vi "WLAN_FrameAnalysis.vi"(8 "error in (no error)":errorcluster, 11 "input cluster":cluster{"t0":dbl, "dt":dbl, "Y":cdb[]}) -> (0 "error out":errorcluster, 1 "Constellation":cdb[](graph), 2 "Modulation parameter":T1, 3 "output bits":i8[](array[numeric]), 4 "Frequency offset":dbl, 5 "SIG valid?":bool)   [LabVIEW 2014]
panel:
  out "size(s) 3":i32
  out "size(s) 2":i32
  out "size(s)":i32
  out "Symbol numbers":i32
  out "encoded bit numbers":u32
  out "original bit numbers":u32
  out "Channel Esitimate":dbl[](graph)
  out "Frequency offset corrected signal":cluster{"t0":dbl, "dt":dbl, "Y":dbl[]}(graph)
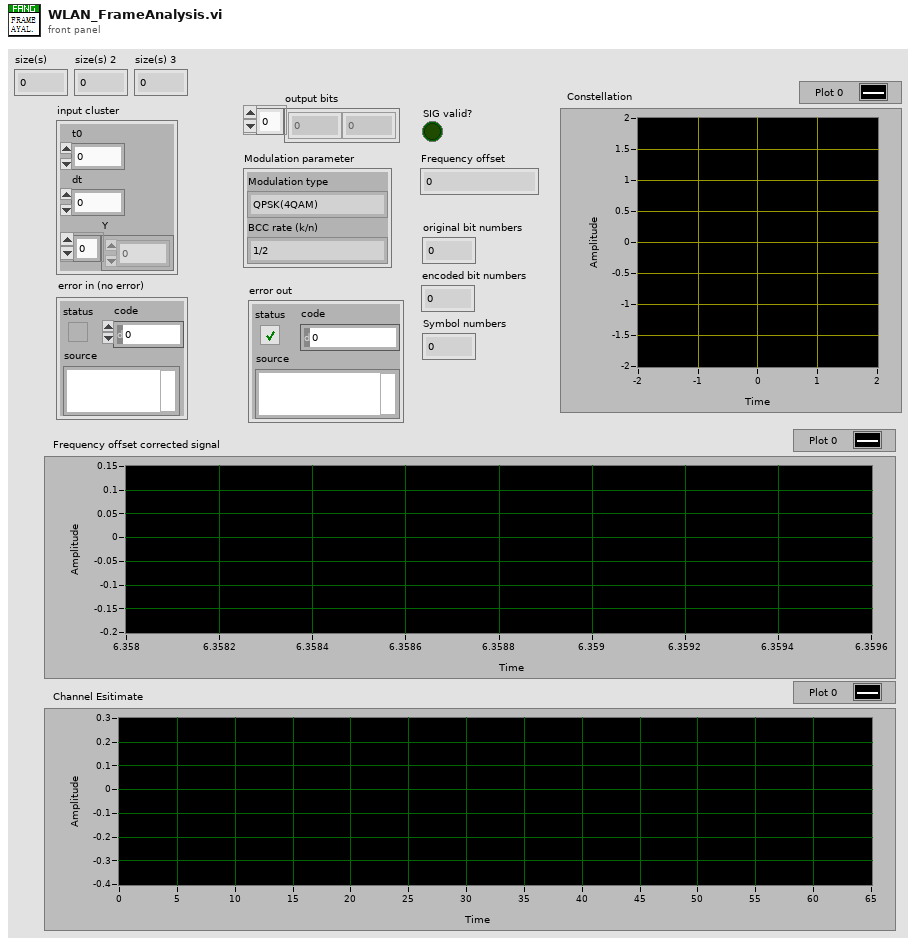
[diagram p1: front panel]
types:
  T1 = cluster{"Modulation type":enum16{"QPSK(4QAM)", "64QAM", "16QAM", "BPSK"}, "BCC rate (k/n)":enum16{"1/2", "2/3", "3/4"}}
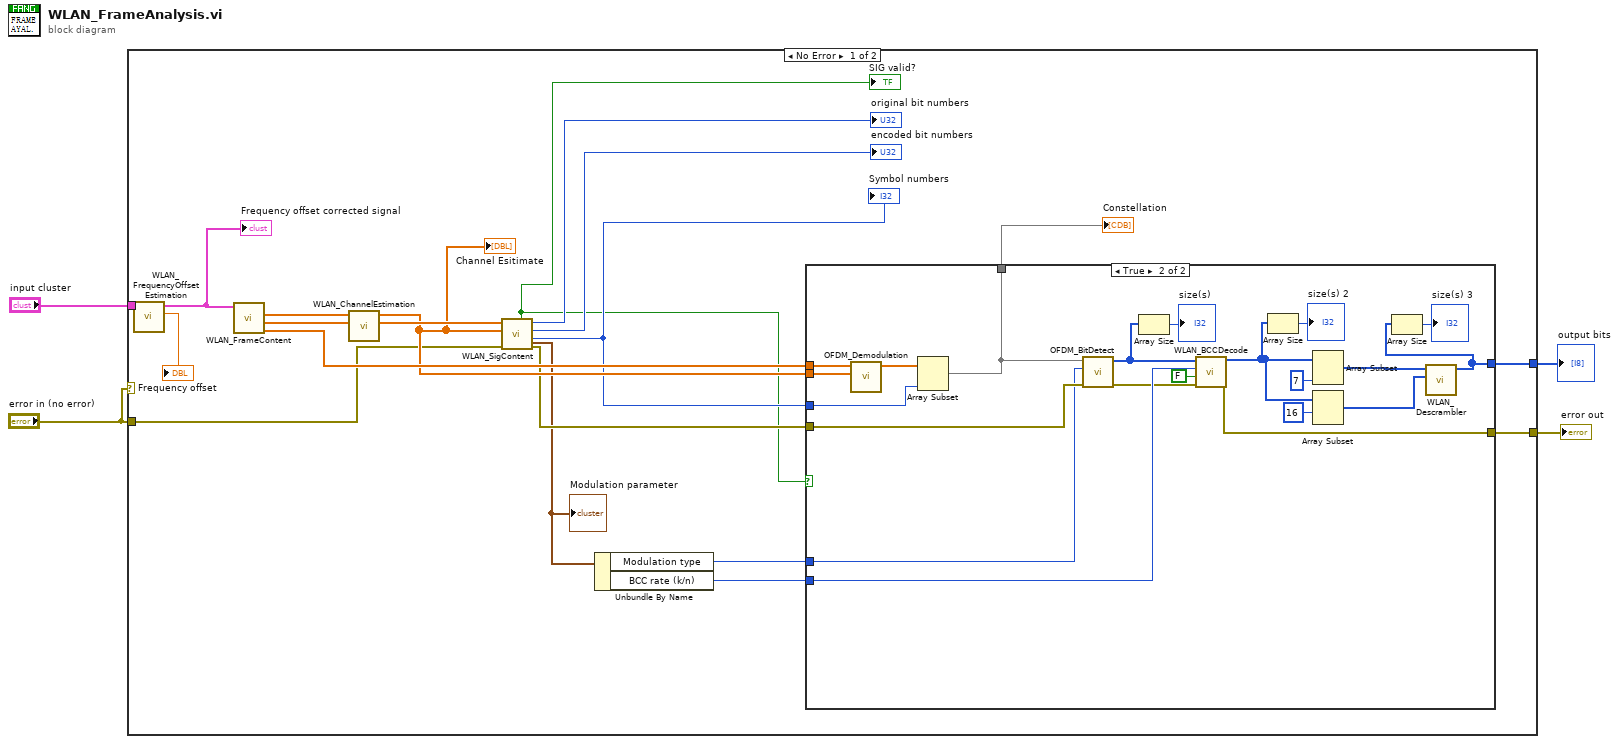
[diagram p0: block diagram]
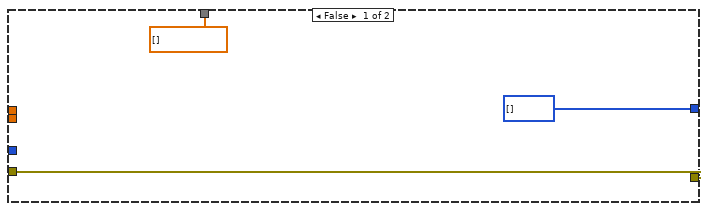
[diagram p2: hidden frame]
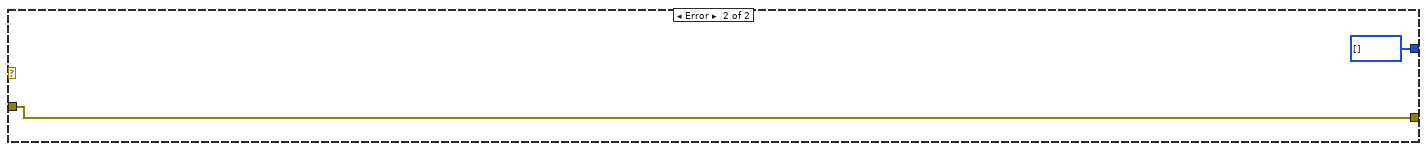
[diagram p3: hidden frame]
diagram:
  n1 = case shown="No Error" "error in (no error)" {
    tunnel: "error in (no error)" -> [w13 w49]
    tunnel: "input cluster" -> [w12 _]
    tunnel: [w11 w49] -> w3
    tunnel: [w10 i8[] [] ("scrambled bits")] -> w2
    frame No Error {
      n2 = call "WLAN_FrequencyOffsetEstimation.vi"("output cluster"=w12) -> ("Frequency offset"=→"Frequency offset":dbl, "output cluster 2"=w20:cluster{"t0":dbl, "dt":dbl, "Y":cdb[]})  [unwired: 8 in]
      "Frequency offset corrected signal" <- w20
      n3 = call "WLAN_FrameContent.vi"("Input cluster"=w20) -> ("DATA"=w23:cdb[], "SIG"=w19:cdb[], "LTF"=w22:cdb[])  [unwired: 7 in, 1 out]
      n4 = call "WLAN_ChannelEstimation.vi"("LTF"=w22) -> ("Frequency estimation"=w18:cdb[])  [unwired: 10 in]
      "Channel Esitimate" <- w18
      n5 = call "WLAN_SigContent.vi"("error in (no error)"=w13, "Frequency channel estimation"=w18, "SIG"=w19) -> ("error out"=w17:errorcluster, "Symbol numbers"=w14:i32, "encoded bit numbers"=→"encoded bit numbers":u32, "original bit numbers"=→"original bit numbers":u32, "Modulation parameter"=w9:T1, "SIG valid?"=w5:bool)  [unwired: 3 in]
      "Modulation parameter" <- w9
      "Symbol numbers" <- w14
      "SIG valid?" <- w5
      n6 = Unbundle By Name(w9) -> ("Modulation type"=w8:enum16{"QPSK(4QAM)", "64QAM", "16QAM", "BPSK"}, "BCC rate (k/n)"=w7:enum16{"1/2", "2/3", "3/4"})
      n7 = case shown="True" w5 {
        tunnel: w23 -> [_ w47]
        tunnel: [w26 w39] -> w11
        tunnel: w18 -> [_ w45]
        tunnel: w17 -> [w26 w44]
        tunnel: w14 -> [_ w43]
        tunnel: w8 -> [_ w42]
        tunnel: [i8[] [] ("scrambled bits") w27] -> w10
        tunnel: w7 -> [_ w41]
        tunnel: [cdb[] [] w33] -> w6
        frame False {
        }
        frame True {
          n8 = call "OFDM_Demodulation.vi"("Frequency channel estimation"=w45, "Input sequence"=w47) -> ("Output sequence"=w46:cdb[])  [unwired: 9 in]
          n9 = Array Subset(array=w46, length=w43) -> (w33:cdb[])  [unwired: 1 in]
          n10 = call "OFDM_BitDetect.vi"("Input symbols"=w33, "Modulation type"=w42, "error in (no error)"=w44) -> ("Output bits"=w32:i8[], "error out"=w40:errorcluster)  [unwired: 6 in]
          n11 = Array Size(array=w32) -> (size(s)=→"size(s)":i32)
          n12 = call "WLAN_BCCDecode.vi"("error in (no error)"=w40, "need add zeros?"=FALSE, "BCC rate (k/n)"=w41, "input bit stream"=w32) -> ("error out"=w39:errorcluster, "output bit stream"=w29:i8[])  [unwired: 6 in]
          n13 = Array Size(array=w29) -> (size(s)=→"size(s) 2":i32)
          n14 = Array Subset(array=w29, length=7) -> (w35:i8[])  [unwired: 1 in]
          n15 = Array Subset(array=w29, index=16) -> (w36:i8[])  [unwired: 1 in]
          n16 = call "WLAN_Descrambler.vi"("scrambler initial bits"=w35, "data bits"=w36) -> ("scrambled bits"=w27:i8[])  [unwired: 7 in]
          n17 = Array Size(array=w27) -> (size(s)=→"size(s) 3":i32)
        }
      }
      "Constellation" <- w6
    }
    frame Error {
    }
  }
  "error out" <- w3
  "output bits" <- w2
